vi "Load_STS_Grid_Param_SubVi.vi"(10 "data":T1(array[cluster]), 11 "STS Param List":u16) -> (3 "Name":string)   [LabVIEW 2014]
uses:
  <userlib>/Nanonis Prog Interface V5/Nanonis Prog Interface.lvlib
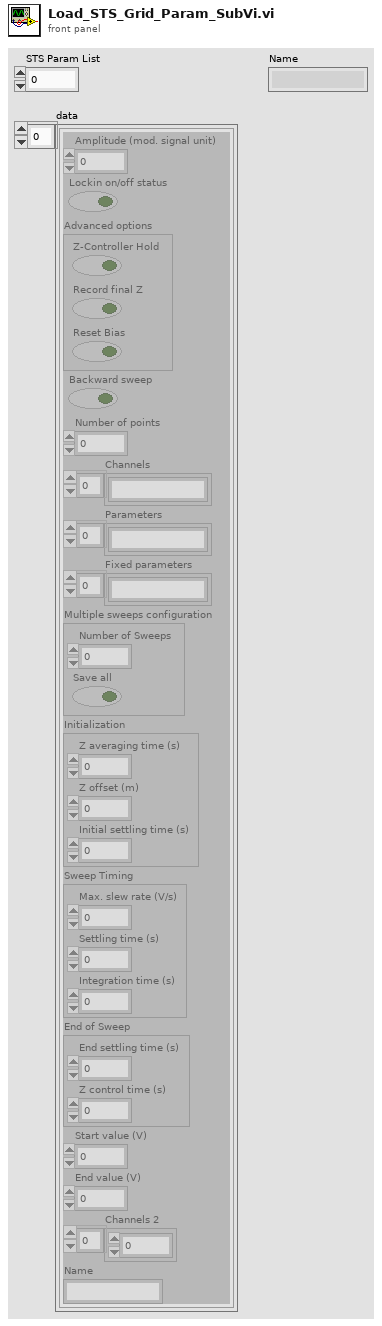
[diagram p1: front panel]
types:
  T1 = cluster{"Amplitude (mod. signal unit)":sgl, "Lockin on/off status":bool, "Advanced options":cluster{"Z-Controller Hold":bool, "Record final Z":bool, "Reset Bias":bool}, "Backward sweep":bool, "Number of points":i32, "Channels":string[], "Parameters":string[], "Fixed parameters":string[], "Multiple sweeps configuration":cluster{"Number of Sweeps":i32, "Save all":bool}, "Initialization":cluster{"Z averaging time (s)":sgl, "Z offset (m)":sgl, "Initial settling time (s)":sgl}, "Sweep Timing":cluster{"Max. slew rate (V/s)":sgl, "Settling time (s)":sgl, "Integration time (s)":sgl}, "End of Sweep":cluster{"End settling time (s)":sgl, "Z control time (s)":sgl}, "Start value (V)":sgl, "End value (V)":sgl, "Channels 2":i32[], "Name":string}[]
  T2 = cluster{"Save all":enum16{"no change", "on", "off"}, "Number of Sweeps (0=no change)":i32}
  T3 = cluster{"Amplitude (mod. signal unit)":sgl, "Lockin on/off status":bool, "Advanced options":cluster{"Z-Controller Hold":bool, "Record final Z":bool, "Reset Bias":bool}, "Backward sweep":bool, "Number of points":i32, "Channels":string[], "Parameters":string[], "Fixed parameters":string[], "Multiple sweeps configuration":cluster{"Number of Sweeps":i32, "Save all":bool}, "Initialization":cluster{"Z averaging time (s)":sgl, "Z offset (m)":sgl, "Initial settling time (s)":sgl}, "Sweep Timing":cluster{"Max. slew rate (V/s)":sgl, "Settling time (s)":sgl, "Integration time (s)":sgl}, "End of Sweep":cluster{"End settling time (s)":sgl, "Z control time (s)":sgl}, "Start value (V)":sgl, "End value (V)":sgl, "Channels 2":i32[], "Name":string}
  T4 = cluster{"Z-Controller Hold":bool, "Record final Z":bool, "Reset Bias":bool}
  T5 = cluster{"Z averaging time (s)":sgl, "Z offset (m)":sgl, "Initial settling time (s)":sgl}
  T6 = cluster{"Max. slew rate (V/s)":sgl, "Settling time (s)":sgl, "Integration time (s)":sgl}
  T7 = cluster{"End settling time (s)":sgl, "Z control time (s)":sgl}
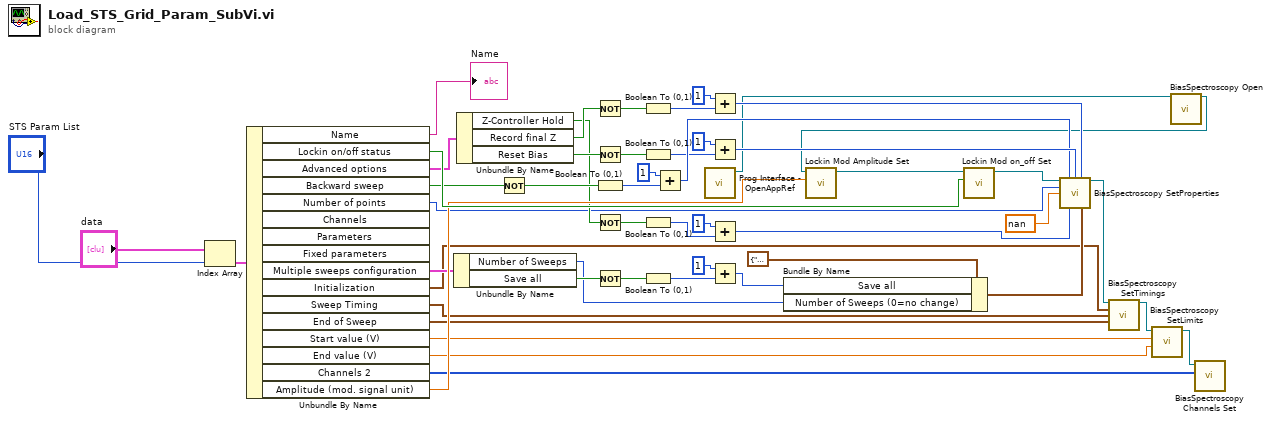
[diagram p0: block diagram]
diagram:
  n1 = Index Array(array="data", index="STS Param List") -> (element=w5:T3)
  n2 = Unbundle By Name(w5) -> ("Name"=→"Name":string, "Lockin on/off status"=w50:bool, "Advanced options"=w17:T4, "Backward sweep"=w18:bool, "Number of points"=w15:i32, "Multiple sweeps configuration"=w16:cluster{"Number of Sweeps":i32, "Save all":bool}, "Initialization"=w14:T5, "Sweep Timing"=w13:T6, "End of Sweep"=w12:T7, "Start value (V)"=w10:sgl, "End value (V)"=w11:sgl, "Channels 2"=w9:i32[], "Amplitude (mod. signal unit)"=w40:sgl)  [unwired: 3 out]
  n3 = Unbundle By Name(w16) -> ("Number of Sweeps"=w30:i32, "Save all"=w34:bool)
  n4 = Unbundle By Name(w17) -> ("Z-Controller Hold"=w25:bool, "Record final Z"=w26:bool, "Reset Bias"=w29:bool)
  n5 = Not(x=w18) -> (.not. x?=w37:bool)
  n6 = Not(x=w26) -> (.not. x?=w35:bool)
  n7 = Not(x=w29) -> (.not. x?=w36:bool)
  n8 = Boolean To (0,1)(Boolean=w37) -> (0, 1=w19:i16)
  n9 = Not(x=w25) -> (.not. x?=w38:bool)
  n10 = Not(x=w34) -> (.not. x?=w39:bool)
  n11 = Boolean To (0,1)(Boolean=w35) -> (0, 1=w21:i16)
  n12 = Boolean To (0,1)(Boolean=w36) -> (0, 1=w27:i16)
  n13 = Boolean To (0,1)(Boolean=w38) -> (0, 1=w23:i16)
  n14 = Boolean To (0,1)(Boolean=w39) -> (0, 1=w31:i16)
  n15 = Add(x=i16 1, y=w19) -> (x+y=w41:i16)
  n16 = call <userlib>:"Prog Interface - OpenAppRef.vi"() -> ("Application reference"=w2:refnum<vi>)  [unwired: 6 in, 1 out]
  n17 = Add(x=i16 1, y=w21) -> (x+y=w48:i16)
  n18 = Add(x=i16 1, y=w27) -> (x+y=w44:i16)
  n19 = Add(x=i16 1, y=w23) -> (x+y=w49:i16)
  n20 = Add(x=i16 1, y=w31) -> (x+y=w33:i16)
  n21 = Bundle By Name(cluster=T2 {"Save all"=enum."no change", "Number of Sweeps (0=no change)"=0} ("Multiple sweeps config"), "Save all"=w33, "Number of Sweeps (0=no change)"=w30) -> (w46:T2)
  n22 = call <userlib>:"BiasSpectroscopy Open.vi"("Application ref in"=w2) -> ("Application ref out"=w1:refnum<vi>)  [unwired: 13 in, 1 out]
  n23 = call <userlib>:"Lockin Mod Amplitude Set.vi"("Amplitude (mod. signal unit)"=w40, "Application ref in"=w1) -> ("Application ref out"=w6:refnum<vi>)  [unwired: 8 in, 1 out]
  n24 = call <userlib>:"Lockin Mod on_off Set.vi"("Lockin ON/OFF"=w50, "Application ref in"=w6) -> ("Application ref out"=w42:refnum<vi>)  [unwired: 8 in, 1 out]
  n25 = call <userlib>:"BiasSpectroscopy SetProperties.vi"("Application ref in"=w42, "Backward sweep (no change)"=w41, "Reset Bias (no change)"=w44, "Record final Z position"=w48, "Number of points (0=no change)"=w15, "Z offset (m) (NaN=no change)"=sgl nan, "Z-Controller hold (no change)"=w49, "Multiple sweeps config"=w46) -> ("Application ref out"=w43:refnum<vi>)  [unwired: 6 in, 1 out]
  n26 = call <userlib>:"BiasSpectroscopy SetTimings.vi"("Application ref in"=w43, "Initialization (NaN)"=w14, "Sweep Timing (NaN)"=w13, "End of Sweep (NaN)"=w12) -> ("Application ref out"=w7:refnum<vi>)  [unwired: 10 in, 1 out]
  n27 = call <userlib>:"BiasSpectroscopy SetLimits.vi"("End value (V)"=w11, "Start value (V)"=w10, "Application ref in"=w7) -> ("Application ref out"=w8:refnum<vi>)  [unwired: 5 in, 1 out]
  n28 = call <userlib>:"BiasSpectroscopy Channels Set.vi"("Channels"=w9, "Application ref in"=w8) -> ()  [unwired: 8 in, 2 out]
